vi "Poition Set Left Right Values.vi"(7 "Left Right PID Values":T1, 8 "Error":errorcluster, 10 "Relative Fwd Back Postion(in)":dbl, 11 "RobotDriveDevRef":T2) -> (0 "Error Out":errorcluster, 3 "RobotDriveDevRef Out":T2)   [LabVIEW 2017, in "WCDrive2018.lvlib"]
uses:
  WCDrive2018.lvlib
  <vilib>/Rock Robotics/WPI/RobotDrive/WPI_RobotDriveMotorSelectorEnum.ctl
  <vilib>/Rock Robotics/SystemInterfaces/DIO/FPGA_DIOPWMChannel.ctl
  <vilib>/Rock Robotics/WPI/PWM/WPI_PWMDeadband.ctl
  <vilib>/Rock Robotics/WPI/MotorControl/WPI_MotorControlType.ctl
  <vilib>/Rock Robotics/WPI/MotorControl/WPI_MotorControlDeviceRef.ctl
  <vilib>/Rock Robotics/WPI/RobotDrive/WPI_RobotDriveDevRef.ctl
  ProtoType Code/EXAMPLE 2017 competition code/roboRIO Code/TypeDefs/Cluster_SRX PID Values.ctl
  <vilib>/Rock Robotics/SystemInterfaces/DIO/FPGA_DIOChannel.ctl
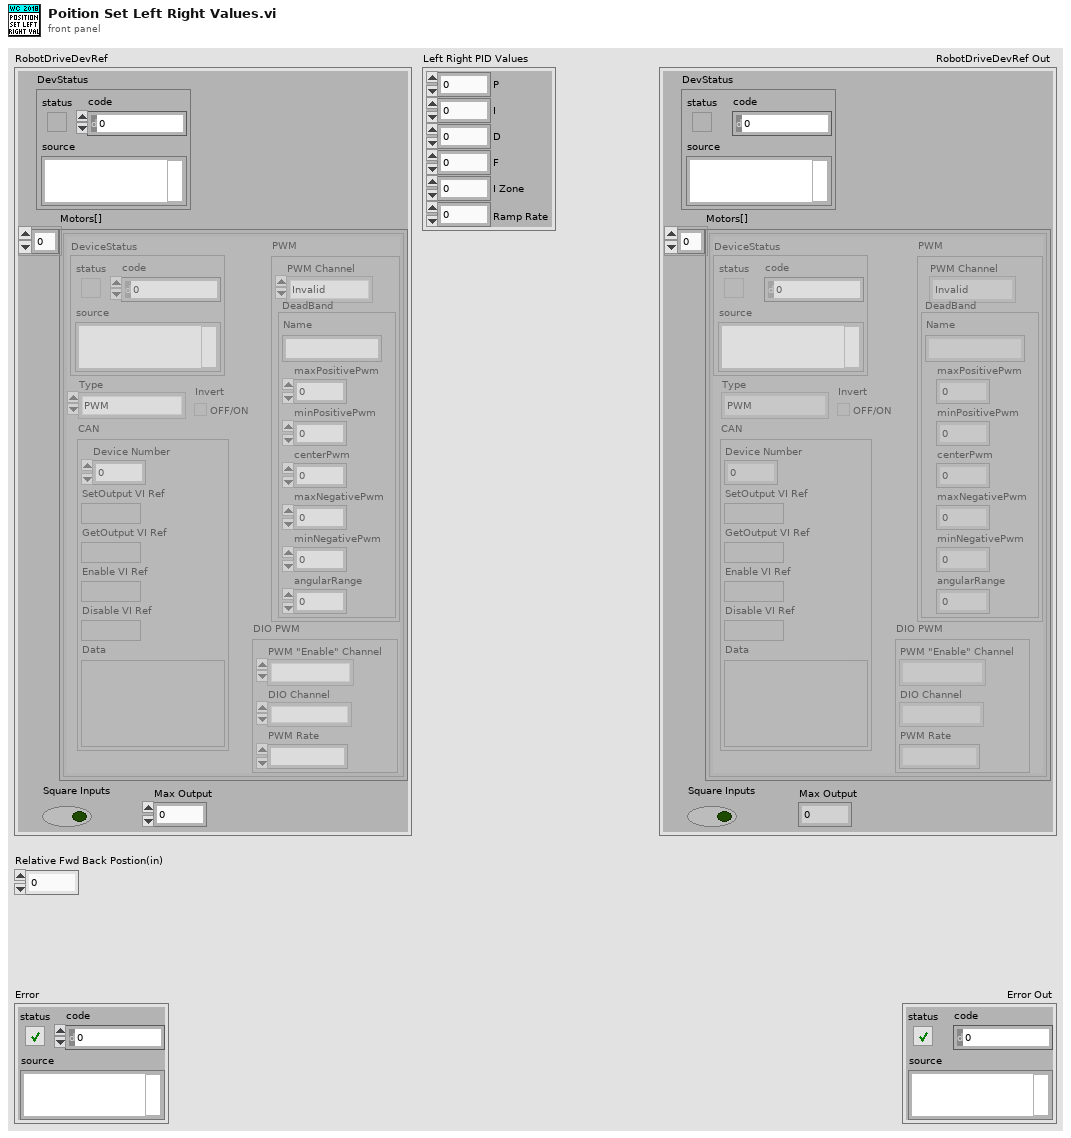
[diagram p1: front panel]
types:
  T1 = typedef "Cluster_SRX PID Values.ctl" = cluster{"P":dbl, "I":dbl, "D":dbl, "F":dbl, "I Zone":dbl, "Ramp Rate":dbl}
  T2 = typedef "WPI_RobotDriveDevRef.ctl" = cluster{"DevStatus":errorcluster, "Motors[]":T3[], "Square Inputs":bool, "Max Output":dbl}
  T3 = typedef "WPI_MotorControlDeviceRef.ctl" = cluster{"DeviceStatus":errorcluster, "Type":T4, "PWM":cluster{"PWM Channel":T5, "DeadBand":T6}, "CAN":cluster{"Device Number":u8, "SetOutput VI Ref":variant, "GetOutput VI Ref":variant, "Enable VI Ref":variant, "Disable VI Ref":variant, "Data":variant}, "Invert":bool, "DIO PWM":cluster{"PWM \"Enable\" Channel":T5, "DIOChannel":T7, "PWM Rate":dbl}}
  T4 = typedef "WPI_MotorControlType.ctl" = enum16{"PWM", "CAN", "DIO PWM"}
  T5 = typedef "FPGA_DIOPWMChannel.ctl" = enum8{"PWM 0", "PWM 1", "PWM 2", "PWM 3", "PWM 4", "PWM 5", "PWM 6", "PWM 7", "PWM 8", "PWM 9", "PWM MXP 0", "PWM MXP 1", "PWM MXP 2", "PWM MXP 3", "PWM MXP 4", "PWM MXP 5", "PWM MXP 6", "PWM MXP 7", "PWM MXP 8", "PWM MXP 9", "Invalid"}
  T6 = typedef "WPI_PWMDeadband.ctl" = cluster{"Name":string, "maxPositivePwm":i32, "minPositivePwm":i32, "centerPwm":i32, "maxNegativePwm":i32, "minNegativePwm":i32, "angularRange":u16}
  T7 = typedef "FPGA_DIOChannel.ctl" = enum8{"DIO 0", "DIO 1", "DIO 2", "DIO 3", "DIO 4", "DIO 5", "DIO 6", "DIO 7", "DIO 8", "DIO 9", "DIO MXP 0", "DIO MXP 1", "DIO MXP 2", "DIO MXP 3", "DIO MXP 4", "DIO MXP 5", "DIO MXP 6", "DIO MXP 7", "DIO MXP 8", "DIO MXP 9", "DIO MXP 10", "DIO MXP 11", "DIO MXP 12", "DIO MXP 13", "DIO MXP 14", "DIO MXP 15", "SPI Port CS1", "SPI Port CS2", "SPI Port CS3", "SPI Port MISO", "SPI Port MOSI", "Invalid"}
  T8 = typedef "WPI_RobotDriveMotorSelectorEnum.ctl" = enum16{"Rear Left Motor", "Rear Right Motor", "Front Left Motor", "Front Right Motor"}
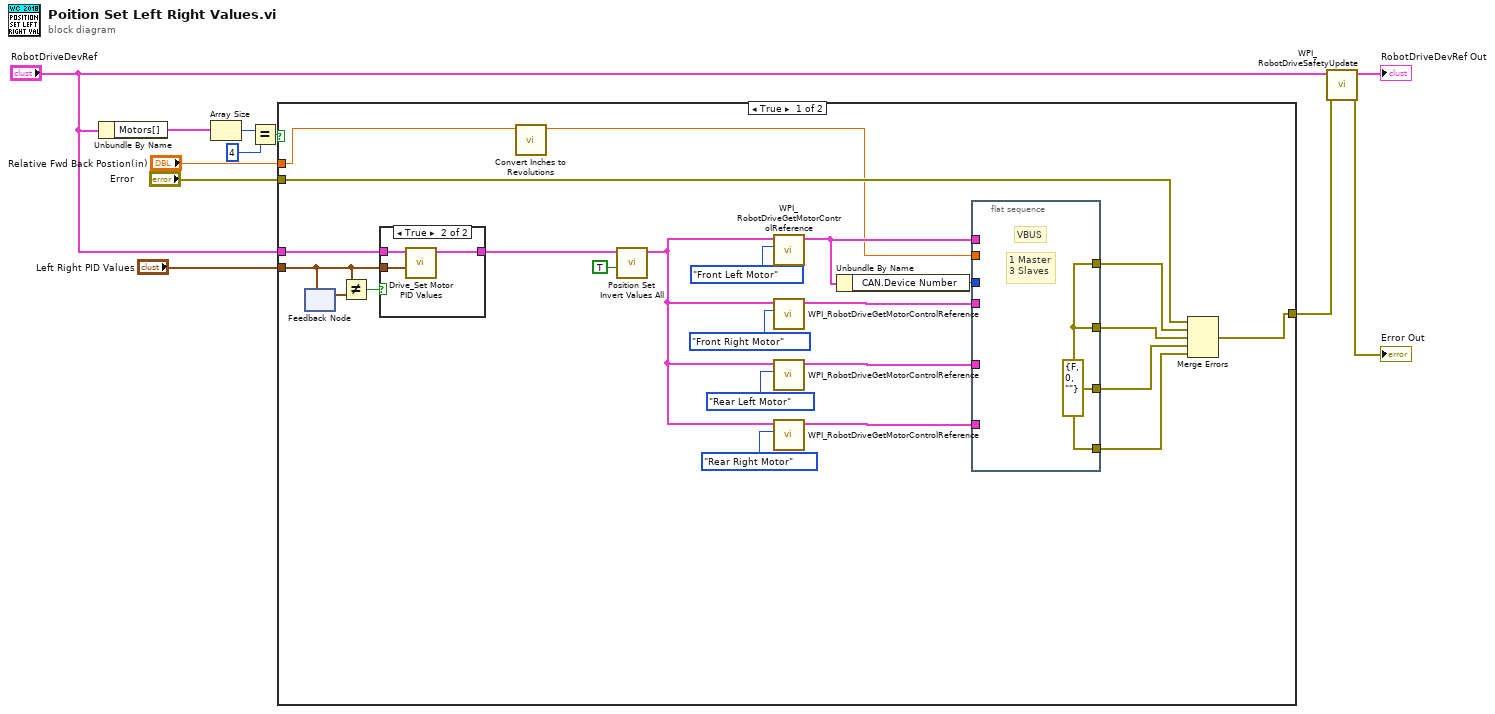
[diagram p0: block diagram]
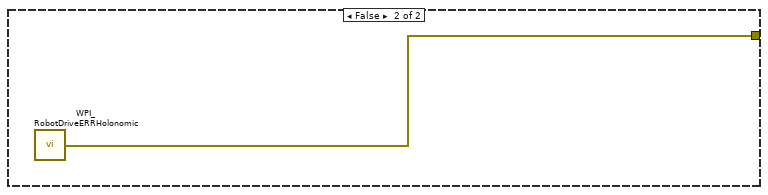
[diagram p3: hidden frame]
diagram:
  n1 = Unbundle By Name("RobotDriveDevRef") -> ("Motors[]"=w8:T3[])
  n2 = Array Size(array=w8) -> (size(s)=w4:i32)
  n3 = Equal?(x=w4, y=4) -> (x = y?=w6:bool)
  n4 = case shown="True" w6 {
    tunnel: "RobotDriveDevRef" -> [w19 _]
    tunnel: [w27 w41] -> w7
    tunnel: "Error" -> [w26 _]
    tunnel: "Relative Fwd Back Postion(in)" -> [w13 _]
    tunnel: "Left Right PID Values" -> [w17 _]
    frame True {
      n5 = feedback-in #1(w17) -> ()
      n6 = feedback #1() -> (w24:T1)  [unwired: 1 in]
      n7 = Not Equal?(x=w17, y=w24) -> (x != y?=w18:bool)
      n8 = case shown="True" w18 {
        tunnel: w19 -> [w37 w40]
        tunnel: [w37 w39] -> w16
        tunnel: w17 -> [_ w38]
        frame False {
        }
        frame True {
          n9 = call "Drive_Set Motor PID Values.vi"("Position Fwd Back PID Values"=w38, "RobotDriveDevRef"=w40) -> ("RobotDriveDevRef Out"=w39:T2)  [unwired: 8 in, 1 out]
        }
      }
      n10 = call "Convert Inches to Revolutions.vi"("Postion(in)"=w13) -> ("Revolutions"=w12:dbl)  [unwired: 10 in]
      n11 = call "Position Set Invert Values All.vi"("FwdBk(F) LR(T)"=TRUE, "RobotDriveDevRef"=w16) -> ("RobotDriveDevRef Out"=w15:T2)  [unwired: 8 in, 1 out]
      n12 = call <vilib>:"WPI_RobotDriveGetMotorControlReference.vi"("MotorIndex"=WPI_RobotDriveMotorSelectorEnum."Front Left Motor", "RobotDriveDevRef"=w15) -> ("MotorControlDeviceRef"=w22:T3)  [unwired: 9 out]
      n13 = call <vilib>:"WPI_RobotDriveGetMotorControlReference.vi"("MotorIndex"=WPI_RobotDriveMotorSelectorEnum."Front Right Motor", "RobotDriveDevRef"=w15) -> ("MotorControlDeviceRef"=w21:T3)  [unwired: 9 out]
      n14 = call <vilib>:"WPI_RobotDriveGetMotorControlReference.vi"("MotorIndex"=WPI_RobotDriveMotorSelectorEnum."Rear Left Motor", "RobotDriveDevRef"=w15) -> ("MotorControlDeviceRef"=w20:T3)  [unwired: 9 out]
      n15 = call <vilib>:"WPI_RobotDriveGetMotorControlReference.vi"("MotorIndex"=WPI_RobotDriveMotorSelectorEnum."Rear Right Motor", "RobotDriveDevRef"=w15) -> ("MotorControlDeviceRef"=w23:T3)  [unwired: 9 out]
      n16 = Unbundle By Name(w22) -> ("CAN.Device Number"=w25:u8)
      n17 = flat-sequence {
        tunnel: [w36] -> w31
        tunnel: [w36] -> w30
        tunnel: [w36] -> w29
        tunnel: [w36] -> w28
        tunnel: w25 -> [_]
        tunnel: w23 -> [_]
        tunnel: w22 -> [_]
        tunnel: w21 -> [_]
        tunnel: w20 -> [_]
        tunnel: w12 -> [_]
        frame #0 {
          w36 = errorcluster {"status"=FALSE, "code"=0, "source"=""} ("error out")
          # "1 Master\n3 Slaves"
          # "VBUS"
        }
      }
      n18 = Merge Errors(w26, w28, w29, w30, w31) -> (w27:errorcluster)
    }
    frame False {
      n19 = call <vilib>:"WPI_RobotDriveERRHolonomic.vi"() -> ("error out"=w41:errorcluster)
    }
  }
  n20 = call <vilib>:"WPI_RobotDriveSafetyUpdate.vi"("error in (no error)"=w7, "RobotDriveDevRef"="RobotDriveDevRef") -> ("error out"=→"Error Out":errorcluster, "RobotDriveDevRef"=→"RobotDriveDevRef Out":T2)  [unwired: 8 out]
